vi "ShouldFlipAcceleration.vi"(11 "Config":T1) -> (3 "Flip?":bool)   [LabVIEW 2017]
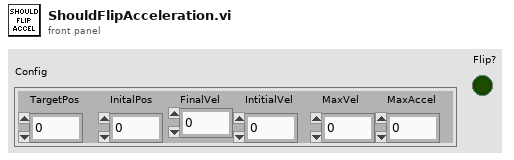
[diagram p1: front panel]
types:
  T1 = cluster{"TargetPos":dbl, "InitalPos":dbl, "FinalVel":dbl, "IntitialVel":dbl, "MaxVel":dbl, "MaxAccel":dbl}
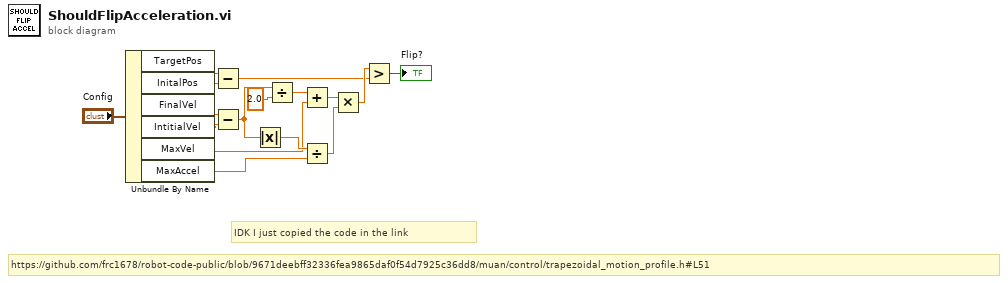
[diagram p0: block diagram]
diagram:
  # "IDK I just copied the code in the link"
  # "https://github.com/frc1678/robot-code-public/blob/9671deebff32336fea9865daf0f54d7925c36dd8/muan/control/trapezoidal_motion_profile.h#L51"
  n1 = Unbundle By Name("Config") -> ("TargetPos"=w13:dbl, "InitalPos"=w14:dbl, "FinalVel"=w12:dbl, "IntitialVel"=w6:dbl, "MaxAccel"=w10:dbl)  [unwired: 1 out]
  n2 = Subtract(x=w13, y=w14) -> (x-y=w2:dbl)
  n3 = Subtract(x=w12, y=w6) -> (x-y=w9:dbl)
  n4 = Absolute Value(x=w9) -> (abs(x)=w11:dbl)
  n5 = Divide(x=w9, y=2.0) -> (x/y=w7:dbl)
  n6 = Add(x=w7, y=w6) -> (x+y=w5:dbl)
  n7 = Divide(x=w11, y=w10) -> (x/y=w4:dbl)
  n8 = Multiply(x=w5, y=w4) -> (x*y=w3:dbl)
  n9 = Greater?(x=w3, y=w2) -> (0:→"Flip?":bool)
